vi "Disconnect.vi"(8 "error in (no error)":errorcluster, 11 "INetworkWriter in":refnum<class "IStreamWriter.lvclass">) -> (0 "error out":errorcluster, 3 "INetworkWriter out":refnum<class "IStreamWriter.lvclass">)   [LabVIEW 2024, in "IStreamWriter.lvclass"]
uses:
  IStreamWriter.lvclass
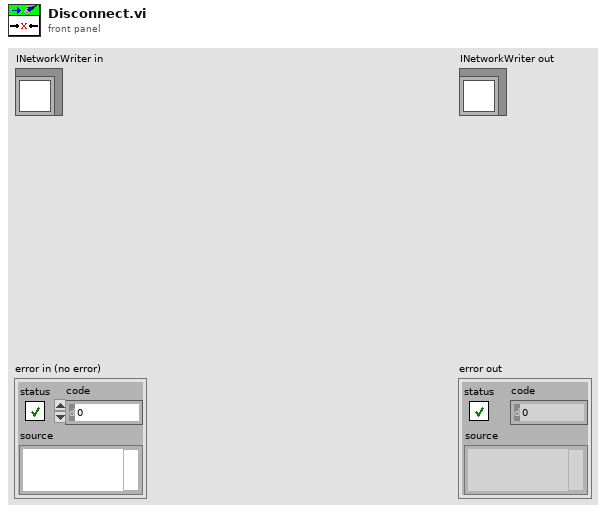
[diagram p1: front panel]
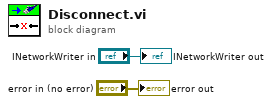
[diagram p0: block diagram]
diagram:
  "error out" <- "error in (no error)"
  "INetworkWriter out" <- "INetworkWriter in"
